vi "Read settings node.vi"(8 "error in (no error)":errorcluster, 9 "Create if necessary? (FALSE)":bool, 10 "Settings node name":string, 11 "CoSy Config File in":refnum<class "CoSy Config File.lvclass">) -> (0 "error out":errorcluster, 1 "Created?":bool, 2 "Settings node":refnum<k20>, 3 "CoSy Config File out":refnum<class "CoSy Config File.lvclass">)   [LabVIEW 2011, in "COSYLib.lvlib" / "CoSy Config File.lvclass"]
doc: "Retrieve a refnum to a <B>settings node</B> (a node directly under the root node).\nIf <B>Create if necessary?</B> is TRUE, the settings node will be created automatically if it doesn't exist yet."
uses:
  CoSy Config File.lvclass
  CoSy Config File.lvclass/CoSy Config File.ctl
  <vilib>/xml/Close Reference(Node).vi
  <vilib>/xml/NI_XML.lvlib
  C:/Program Files (x86)/National Instruments/LabVIEW 2011/resource/objmgr/DOMUserDefRef.rc
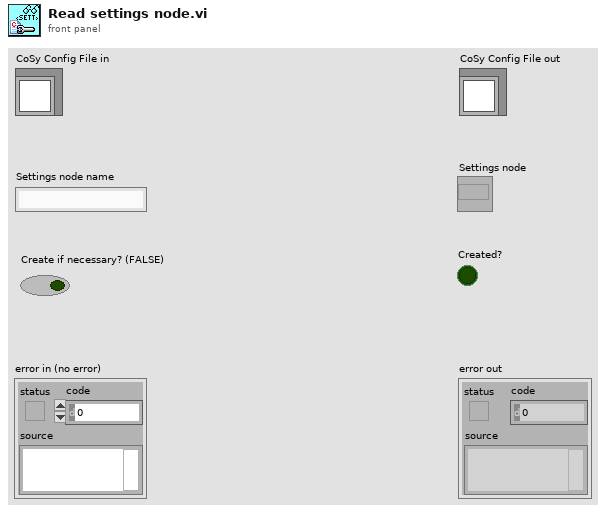
[diagram p1: front panel]
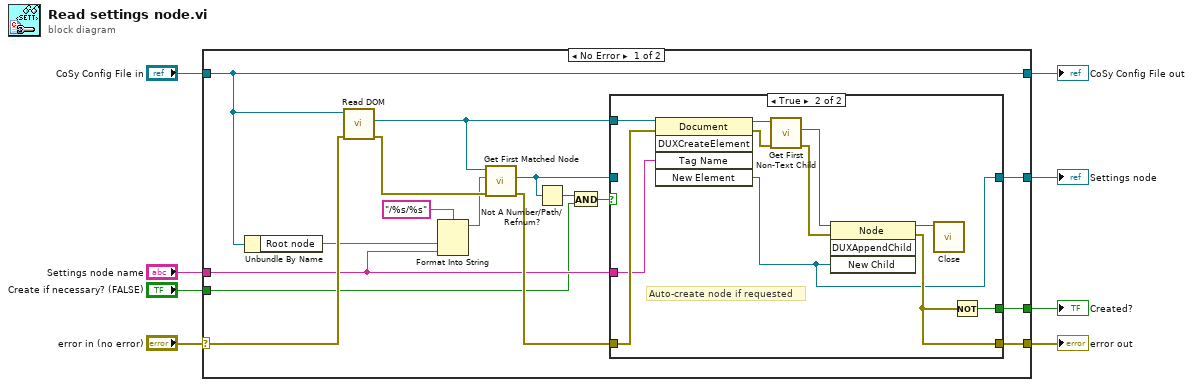
[diagram p0: block diagram]
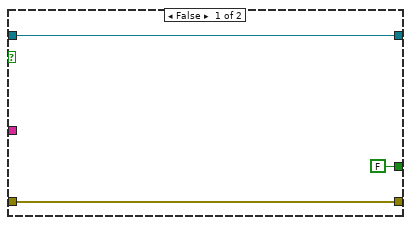
[diagram p2: hidden frame]
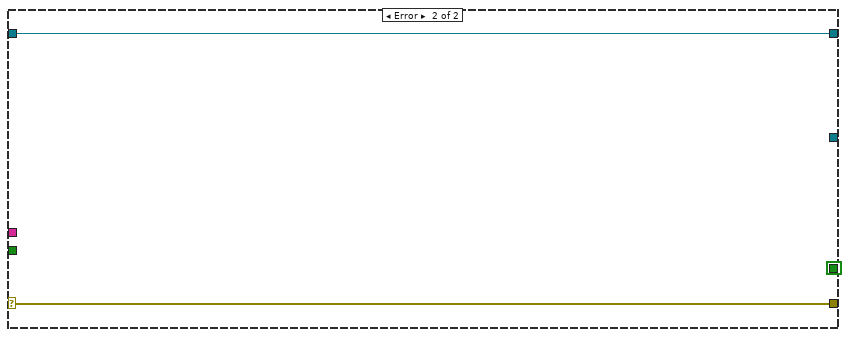
[diagram p3: hidden frame]
diagram:
  n1 = case shown="No Error" "error in (no error)" {
    selector: "error in (no error)" -> [w22 w41]
    tunnel: [w21 w41] -> w7
    tunnel: [w14 w40] -> w5
    tunnel: "CoSy Config File in" -> [w14 w40]
    tunnel: "Settings node name" -> [w12 _]
    tunnel: "Create if necessary? (FALSE)" -> [w11 _]
    tunnel: [w10 _] -> w2
    tunnel: [w9 FALSE] -> w1
    frame No Error {
      n2 = Unbundle By Name(w14) -> ("Root node"=w15:string)
      n3 = call "Read DOM.vi"("error in (no error)"=w22, "CoSy Config File in"=w14) -> ("error out"=w23:errorcluster, "DOM"=w13:refnum<k20>)  [unwired: 7 in, 1 out]
      n4 = Format Into String(format string="/%s/%s", w15, w12) -> (resulting string=w19:string)  [unwired: 2 in, 1 out]
      n5 = call <vilib>:"Get First Matched Node.vi"("error in (no error)"=w23, "XPath expression"=w19, "node in"=w13) -> ("error out"=w24:errorcluster, "node result"=w17:refnum<k20>)  [unwired: 6 in, 1 out]
      n6 = Not A Number/Path/Refnum?(number/path/refnum=w17) -> (NaN/Path/Refnum?=w18:bool)
      n7 = And(x=w18, y=w11) -> (x .and. y?=w16:bool)
      n8 = case shown="True" w16 {
        tunnel: w24 -> [w27 w38]
        tunnel: w13 -> [_ w34]
        tunnel: w12 -> [_ w33]
        tunnel: w17 -> [w26 _]
        tunnel: [w26 w30] -> w10
        tunnel: [w27 w35] -> w21
        tunnel: [FALSE w28] -> w9
        frame False {
        }
        frame True {
          # "Auto-create node if requested"
          n9 = invoke class="Document" method="DUXCreateElement"(reference=w34, error in=w38, "Tag Name"=w33) -> (reference out=w32:refnum<k20>, error out=w37:errorcluster, "New Element"=w30:refnum<k20>)  [unwired: 2 in, 2 out]
          n10 = call <vilib>:"Get First Non-Text Child.vi"("error in (no error)"=w37, "node in"=w32) -> ("error out"=w36:errorcluster, "child node"=w31:refnum<k20>)  [unwired: 6 in, 2 out]
          n11 = invoke class="Node" method="DUXAppendChild"(reference=w31, error in=w36, "New Child"=w30) -> (reference out=w29:refnum<k20>, error out=w35:errorcluster)  [unwired: 1 in, 2 out]
          n12 = call-poly <vilib>:"Close.vi"("node"=w29) -> ()  [unwired: 8 in, 1 out]
          n13 = Not(x=w35) -> (.not. x?=w28:bool)
        }
      }
    }
    frame Error {
    }
  }
  "error out" <- w7
  "CoSy Config File out" <- w5
  "Settings node" <- w2
  "Created?" <- w1
